vi "StartSync.vi"(8 "error in (no error)":errorcluster, 11 "SyncPluginBase":refnum<class "SyncPluginBase.lvclass">) -> (0 "error out":errorcluster, 3 "SyncPluginBase":refnum<class "SyncPluginBase.lvclass">)   [LabVIEW 2014, in "SyncPlugins.lvlib" / "SyncPluginBase.lvclass"]
uses:
  SyncPluginBase.lvclass
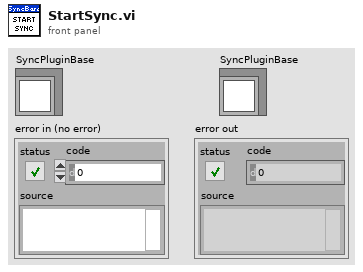
[diagram p1: front panel]
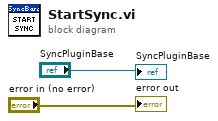
[diagram p0: block diagram]
diagram:
  "SyncPluginBase" <- "SyncPluginBase"
  "error out" <- "error in (no error)"
